vi "Get Form Name.vi"(8 "error in (no error)":errorcluster, 11 "Form Model in":refnum<class "Form Model.lvclass">) -> (0 "error out":errorcluster, 2 "Form ID":T1, 3 "Form Model out":refnum<class "Form Model.lvclass">)   [LabVIEW 2020, in "Form Model.lvlib" / "Form Model.lvclass"]
uses:
  Form Model.lvclass
  Autoclose manager/Form ID.ctl
  Form Model.lvclass/Form Model.ctl
  Form Configuration/Form Model Configuration.lvclass
  Form Server Interfaces.lvlib
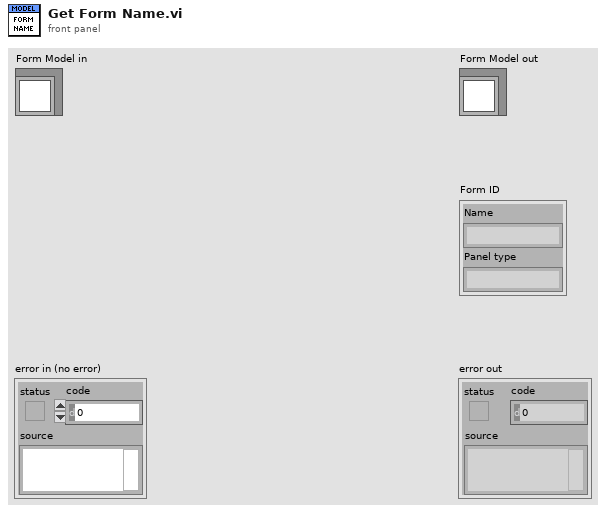
[diagram p1: front panel]
types:
  T1 = typedef "Form Server Interfaces.lvlib/Form ID.ctl" = cluster{"Name":string, "Panel type":string}
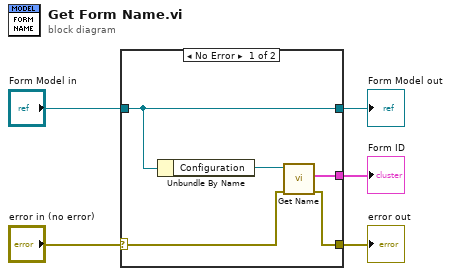
[diagram p0: block diagram]
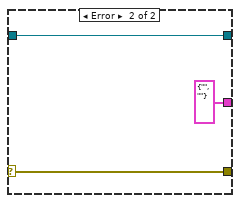
[diagram p2: hidden frame]
diagram:
  n1 = case shown="No Error" "error in (no error)" {
    selector: "error in (no error)" -> [w7 w13]
    tunnel: [w6 w13] -> w4
    tunnel: [w10 w12] -> w2
    tunnel: "Form Model in" -> [w10 w12]
    tunnel: [w8 T1 {"Name"="", "Panel type"=""} ("Form ID")] -> w1
    frame No Error {
      n2 = Unbundle By Name(w10) -> ("Configuration"=w9:refnum<class "Form Model Configuration.lvclass">)
      n3 = call-dynamic "Get Name.vi"("error in (no error)"=w7, "Form Configuration in"=w9) -> ("error out"=w6:errorcluster, "Form ID"=w8:T1)  [unwired: 7 in, 1 out]
    }
    frame Error {
    }
  }
  "error out" <- w4
  "Form Model out" <- w2
  "Form ID" <- w1
